vi "Set Setpoint.vi"(7 "Select Channel":i32=1 min=1 max=4 step=1, 8 "error in (no error)":errorcluster, 10 "Setpoint":dbl, 11 "Lakeshore 336 in":refnum<class "Lakeshore 336.lvclass">) -> (0 "error out":errorcluster, 3 "Lakeshore 336 out":refnum<class "Lakeshore 336.lvclass">)   [LabVIEW 2022 SP3, in "Lakeshore 336.lvclass"]
uses:
  Lakeshore 336.lvclass
  Lakeshore 336.lvclass/Lakeshore 336.ctl
  Temp Control.lvclass
  <instrlib>/Lake Shore 336/Lake Shore 336.lvlib
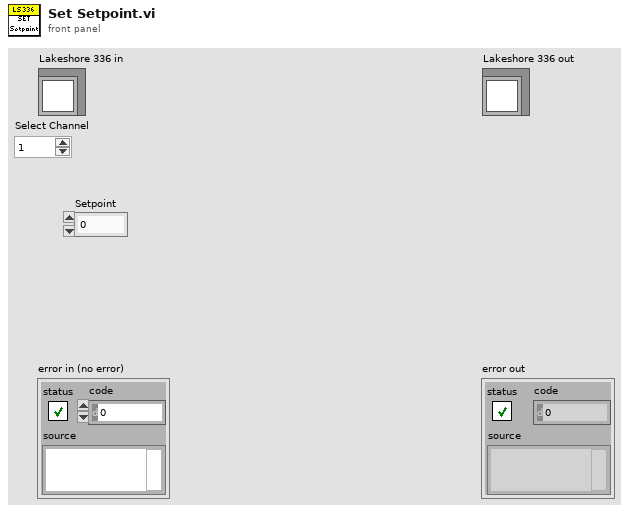
[diagram p1: front panel]
types:
  T1 = typedef "Lakeshore 336.lvclass/Lakeshore 336 Settings cluster.ctl" = cluster{"Lake Shore 336 Address":refnum<visa-resource-name>, "Output Ch":T2[], "Input Ch":T4[], "Prefix":string, "Setpoints":dbl[]}
  T2 = typedef "Lakeshore 336.lvclass/Lakeshore 336 Channel Settings cluster.ctl" = cluster{"Input (0:None)":u16, "Power Up Enable (F: Off)":bool, "Mode (0:Off)":u16, "Max Current (0:User Specified)":u16, "Heater Out Display (1:Current)":u16, "Max User Current (2.000)":dbl, "Heater Resistance (1:25 Ohms)":u16, "PID":T3, "Name":string}
  T3 = typedef "Lakeshore 336.lvclass/Lakeshore 336 PID cluster.ctl" = cluster{"P":dbl, "I":dbl, "D":dbl}
  T4 = typedef "Lakeshore 336.lvclass/Lakeshore 336 Input Ch config cluster.ctl" = cluster{"Name":string}
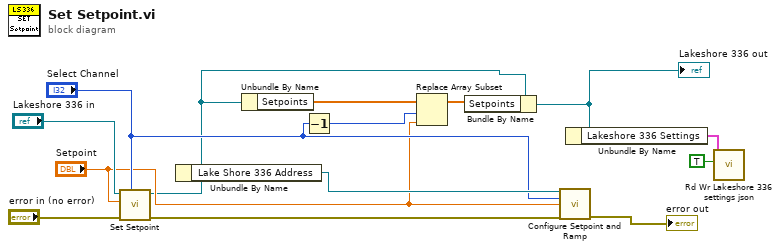
[diagram p0: block diagram]
diagram:
  n1 = call-parent "Set Setpoint.vi"("Select Channel"="Select Channel", "error in (no error)"="error in (no error)", "Setpoint"="Setpoint", "Temp Control in"="Lakeshore 336 in") -> ("error out"=w12:errorcluster, "Temp Control out"=w4:refnum<class "Lakeshore 336.lvclass">)  [unwired: 6 in]
  n2 = Unbundle By Name(w4) -> ("Lake Shore 336 Address"=w11:refnum<visa-resource-name>)
  n3 = Unbundle By Name(w4) -> ("Setpoints"=w9:dbl[])
  n4 = Decrement(x="Select Channel") -> (x-1=w7:i32)
  n5 = Replace Array Subset(array=w9, new element="Setpoint", index=w7) -> (w5:dbl[])
  n6 = Bundle By Name(cluster=w4, "Setpoints"=w5) -> (w3:refnum<class "Lakeshore 336.lvclass">)
  "Lakeshore 336 out" <- w3
  n7 = call <instrlib>:"Configure Setpoint and Ramp.vi"("VISA resource name"=w11, "Output's Control Loop (1:1)"="Select Channel", "Setpoint (0.00000)"="Setpoint", "error in (no error)"=w12) -> ("error out"=→"error out":errorcluster)  [unwired: 10 in, 1 out]
  n8 = Unbundle By Name(w3) -> ("Lakeshore 336 Settings"=w2:T1)
  n9 = call "Rd Wr Lakeshore 336 settings json.vi"("Write? (F:Read)"=TRUE, "Lakeshore 336 Settings"=w2) -> ()  [unwired: 8 in, 2 out]
